vi "Add Block Diagram Content.vi"(8 "error in (no error)":errorcluster, 10 "ModuleLoop":T1, 11 "EST Output in":refnum<class "EST Output.lvclass">) -> (0 "error out":errorcluster, 2 "Term Refnum":refnum<vi>, 3 "EST Output out":refnum<class "EST Output.lvclass">)   [LabVIEW 2015, in "EST Output.lvclass"]
uses:
  EST Output.lvclass
  Loop/Block Diagram/Module.Refs.ctl
  <vilib>/Utility/miscctls.llb/LVPointTypeDef.ctl
  EST Output.lvclass/EST Output.ctl
  IO Class/Read IP Core Path.vi
  IO Class/Read Signal Name.vi
  Loop/Structures/Structures.lvclass
  Loop/Block Diagram/Block Diagram.lvclass
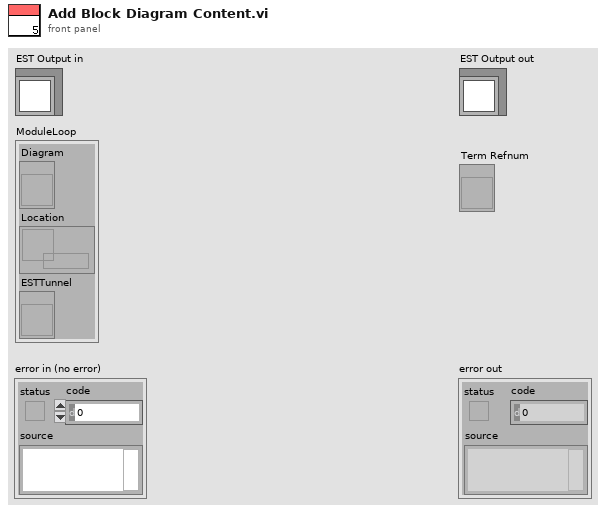
[diagram p1: front panel]
types:
  T1 = typedef "Block Diagram.lvclass/Module.Refs.ctl" = cluster{"Diagram":refnum<vi>, "Location":refnum<data-value>, "ESTTunnel":refnum<vi>}
  T2 = typedef "LVPointTypeDef.ctl" = cluster{"Horizontal":i16, "Vertical":i16}
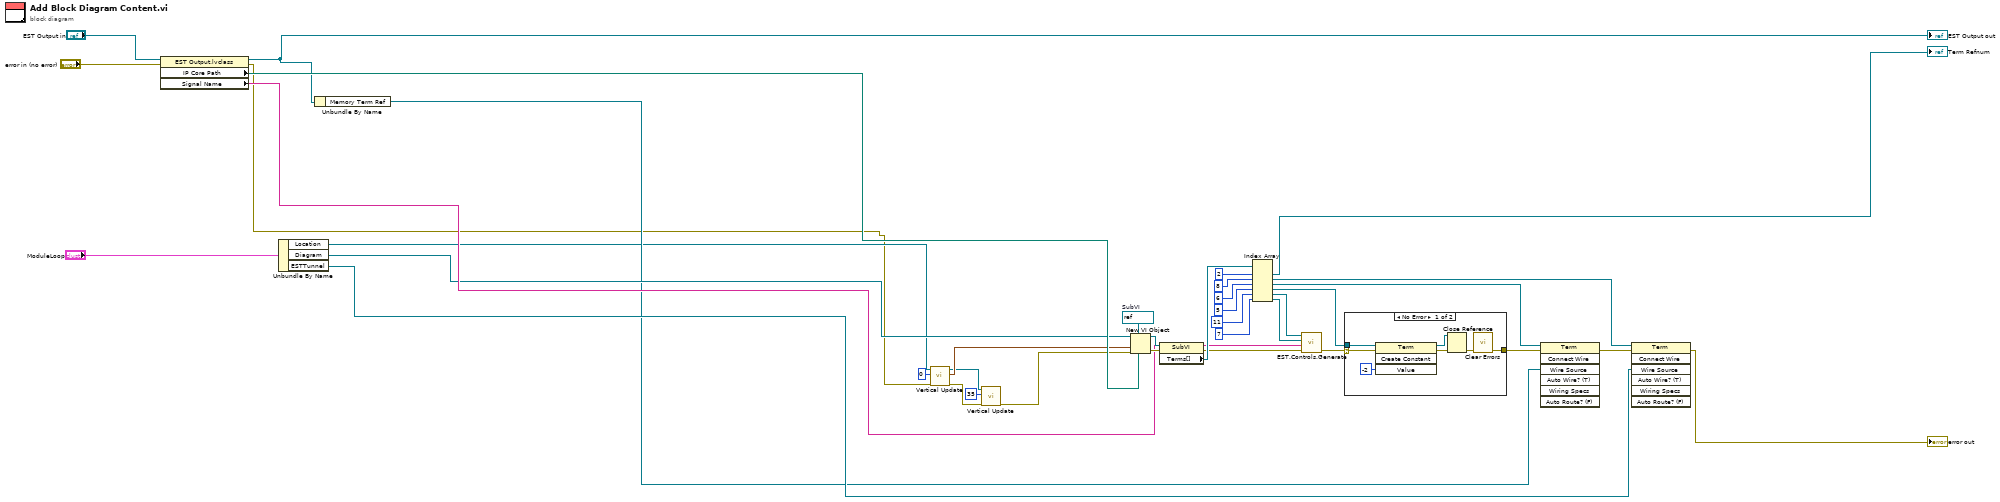
[diagram p0: block diagram]
diagram:
  w33 = refnum<vi> refnum  # SubVI
  n1 = property class="EST Output.lvclass"(reference="EST Output in", error in="error in (no error)") -> (reference out=w9:refnum<class "EST Output.lvclass">, error out=w5:errorcluster, "IP Core Path"=w14:path, "Signal Name"=w15:string)
  "EST Output out" <- w9
  n2 = Unbundle By Name("ModuleLoop") -> ("Location"=w7:refnum<data-value>, "Diagram"=w13:refnum<vi>, "ESTTunnel"=w16:refnum<vi>)
  n3 = Unbundle By Name(w9) -> ("Memory Term Ref"=w12:refnum<vi>)
  n4 = call "Vertical Update.vi"("error in (no error)"=w5, "Vertical Change"=i16 0, "Location"=w7) -> ("error out"=w2:errorcluster, "location out"=w6:T2, "Location"=w3:refnum<data-value>)  [unwired: 6 in]
  n5 = call "Vertical Update.vi"("error in (no error)"=w2, "Vertical Change"=i16 35, "Location"=w3) -> ("error out"=w1:errorcluster)  [unwired: 6 in, 2 out]
  n6 = New VI Object(vi object class=w33, owner refnum=w13, position/next to=w6, 6:w14, 8:w1) -> (object refnum=w36:refnum<vi>, 0:w37:errorcluster)  [unwired: 3 in]
  n7 = property class="SubVI"(reference=w36, error in=w37) -> (error out=w20:errorcluster, "Terms[]"=w34:refnum<vi>[])  [unwired: 1 out]
  n8 = Index Array(array=w34, index #1=2 ("index"), index #2=8 ("index"), index #3=6 ("index"), index #4=5 ("index"), index #5=11 ("index"), index #6=7 ("index")) -> (element #1=→"Term Refnum":refnum<vi>, element #2=w23:refnum<vi>, element #3=w27:refnum<vi>, element #4=w29:refnum<vi>, element #5=w21:refnum<vi>, element #6=w22:refnum<vi>)
  n9 = call "EST.Controls.Generate.vi"("error in (no error)"=w20, "IO Name"=w15, "Input.Ref"=w22, "Settings.Ref"=w21) -> ("error out"=w19:errorcluster)  [unwired: 7 in]
  n10 = case shown="No Error" w19 {
    selector: w19 -> [w43 w46]
    tunnel: w29 -> [w45 _]
    tunnel: [w39 w46] -> w28
    frame No Error {
      n11 = invoke class="Term" method="Create Constant"(reference=w45, error in=w43, "Value"=i8 -2 ("shift")) -> (reference out=w41:refnum<vi>, error out=w42:errorcluster)  [unwired: 1 in, 2 out]
      n12 = Close Reference(reference=w41, error in (no error)=w42) -> (error out=w40:errorcluster)
      n13 = call <vilib>:"Clear Errors.vi"("error in (no error)"=w40) -> ("error out"=w39:errorcluster)  [unwired: 5 in, 1 out]
    }
    frame Error {
    }
  }
  n14 = invoke class="Term" method="Connect Wire"(reference=w27, error in=w28, "Wire Source"=w12) -> (error out=w24:errorcluster)  [unwired: 4 in, 6 out]
  n15 = invoke class="Term" method="Connect Wire"(reference=w23, error in=w24, "Wire Source"=w16) -> (error out=→"error out":errorcluster)  [unwired: 4 in, 6 out]
